vi "Arduino_Comms_Tilt_Table_student.vi"() -> ()   [LabVIEW 2014]
uses:
  <vilib>/Instr/_visa.llb/VISA Configure Serial Port (Instr).vi
panel:
  out "XY Graph":cluster{dbl[], "Buffer Out":sgl[]}[](graph)
  in  "Outer Plate":i8
  in  "Inner Plate":i8
  out "Response":string
  in  "stop":bool
  in  "Arduino Port":refnum<visa-resource-name>="COM9"
  # "Scale (x 0.1deg or x10us)"
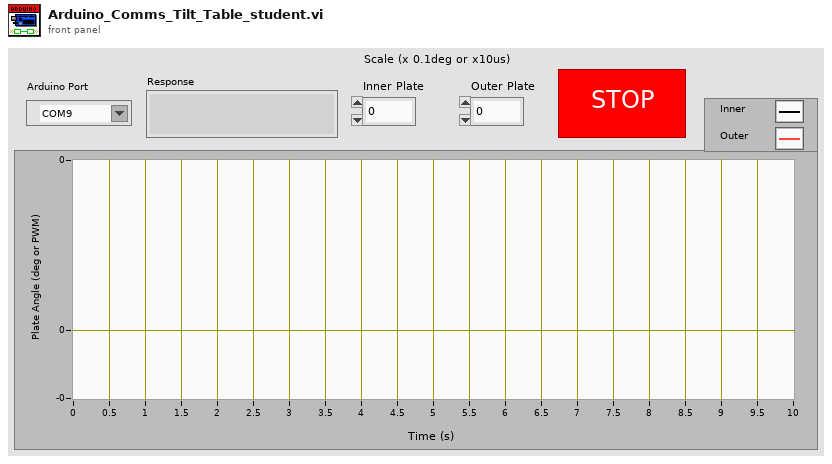
[diagram p1: front panel]
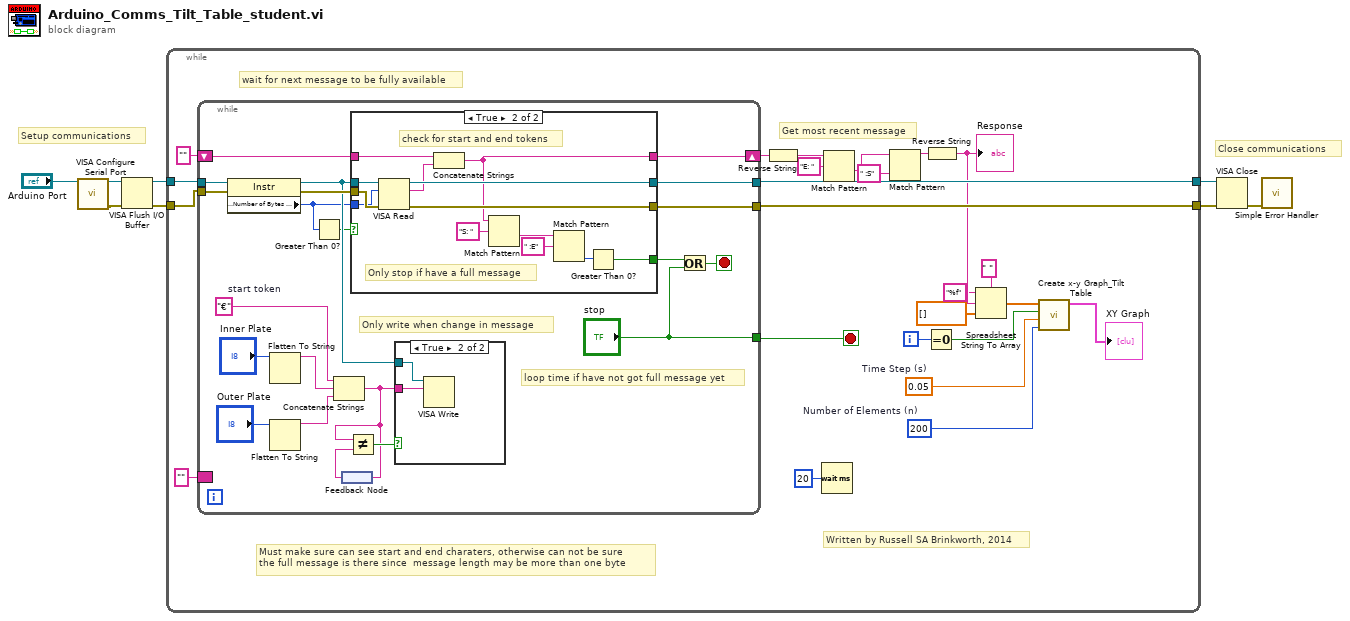
[diagram p0: block diagram]
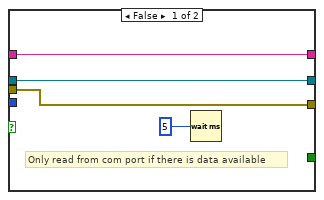
[diagram p3: hidden frame]
diagram:
  # "Close communications"
  # "Setup communications"
  n1 = call-poly "VISA Configure Serial Port"("VISA resource name"="Arduino Port") -> ("VISA resource name out"=w3:refnum<visa-resource-name>, "error out"=w4:errorcluster)  [unwired: 8 in, 5 out]
  n2 = VISA Flush I/O Buffer(VISA resource name=w3, error in (no error)=w4) -> (VISA resource name out=w1:refnum<visa-resource-name>, error out=w2:errorcluster)  [unwired: 1 in]
  n3 = while {
    tunnel: w1 -> [w26]
    tunnel: w2 -> [w31]
    tunnel: [w30] -> w6
    tunnel: [w29] -> w7
    i -> [w13]
    stop <- w27 stop-if-true
    w9 = 200  # Number of Elements (n)
    w10 = 0.05  # Time Step (s)
    # "Written by Russell SA Brinkworth, 2014"
    # "Get most recent message"
    # "Must make sure can see start and end charaters, otherwise can not be sure \nthe full message is there since  message length may be more than one byte"
    # "wait for next message to be fully available"
    n4 = while {
      tunnel: w26 -> [w53]
      tunnel: w31 -> [w52]
      tunnel: [w50] -> w30
      tunnel: [w49] -> w29
      shift-right: [w48] -> w15
      shift-left: "" -> [w47]
      tunnel: ["stop"] -> w27
      border: "" -> [_]
      stop <- w45 stop-if-true
      w40 = "€"  # start token
      # "loop time if have not got full message yet"
      # "Only write when change in message"
      n5 = property class="Instr"(reference=w53, error in=w52) -> (reference out=w43:refnum<visa-resource-name>, error out=w51:errorcluster, "Serial Settings:Number of Bytes at Serial Port"=w38:u32)
      n6 = Flatten To String(anything="Inner Plate") -> (data string=w41:string)  [unwired: 3 in, 2 out]
      n7 = Flatten To String(anything="Outer Plate") -> (data string=w36:string)  [unwired: 3 in, 2 out]
      n8 = Greater Than 0?(x=w38) -> (x > 0?=w39:bool)
      n9 = Concatenate Strings(w40, w41, w36) -> (w33:string)
      n10 = feedback-in #1(w33) -> ()
      n11 = feedback #1() -> (w34:string)
      n12 = Not Equal?(x=w33, y=w34) -> (x != y?=w35:bool)
      n13 = case shown="True" w39 {
        tunnel: w38 -> [_ w70]
        tunnel: w43 -> [w59 w72]
        tunnel: w51 -> [w58 w71]
        tunnel: [w59 w69] -> w50
        tunnel: [w58 w68] -> w49
        tunnel: [_ w67] -> w46
        tunnel: w47 -> [w57 w63]
        tunnel: [w57 w62] -> w48
        frame False {
          # "Only read from com port if there is data available"
          n14 = Wait (ms)(milliseconds to wait=u32 5) -> ()  [unwired: 1 out]
        }
        frame True {
          # "check for start and end tokens"
          # "Only stop if have a full message"
          n15 = VISA Read(VISA resource name=w72, byte count=w70, error in (no error)=w71) -> (VISA resource name out=w69:refnum<visa-resource-name>, read buffer=w64:string, error out=w68:errorcluster)  [unwired: 1 out]
          n16 = Concatenate Strings(w63, w64) -> (w62:string)
          n17 = Match Pattern(string=w62, regular expression="S: ") -> (after substring=w65:string)  [unwired: 1 in, 3 out]
          n18 = Match Pattern(string=w65, regular expression=" :E") -> (offset past match=w66:i32)  [unwired: 1 in, 3 out]
          n19 = Greater Than 0?(x=w66) -> (x > 0?=w67:bool)
        }
      }
      n20 = case shown="True" w35 {
        tunnel: w43 -> [_ w55]
        tunnel: w33 -> [_ w54]
        frame False {
        }
        frame True {
          n21 = VISA Write(VISA resource name=w55, write buffer=w54) -> ()  [unwired: 1 in, 3 out]
        }
      }
      n22 = Or(x=w46, y="stop") -> (x .or. y?=w45:bool)
    }
    n23 = Reverse String(1:w15) -> (0:w25:string)
    n24 = Wait (ms)(milliseconds to wait=u32 20) -> ()  [unwired: 1 out]
    n25 = Match Pattern(string=w25, regular expression="E: ") -> (after substring=w21:string)  [unwired: 1 in, 3 out]
    n26 = Match Pattern(string=w21, regular expression=" :S") -> (before substring=w22:string)  [unwired: 1 in, 3 out]
    n27 = Equal To 0?(x=w13) -> (x = 0?=w12:bool)
    n28 = Reverse String(1:w22) -> (0:w19:string)
    "Response" <- w19
    n29 = Spreadsheet String To Array(delimiter (Tab)=" ", format string="%f", spreadsheet string=w19, array type (2D Dbl)=dbl[] []) -> (array=w14:dbl[])
    n30 = call "Create x-y Graph_Tilt Table.vi"("Number of Elements (n)"=w9, "Time Step (s)"=w10, "Reset"=w12, "Data In"=w14) -> ("XY Graph"=→"XY Graph":cluster{dbl[], "Buffer Out":sgl[]}[])  [unwired: 7 in]
  }
  n31 = VISA Close(VISA resource name=w6, error in (no error)=w7) -> (error out=w5:errorcluster)
  n32 = call <vilib>:"Simple Error Handler.vi"("error in (no error)"=w5) -> ()  [unwired: 1 in, 8 out]
